vi "SCCSup OpenCloseFP.vi"(7 "function":enum16{"open FP", "close FP"}(ring), 8 "error in (no error)":errorcluster, 11 "VI Refnum in":refnum<vi>) -> (0 "error out":errorcluster, 3 "VI Refnum out":refnum<vi>)   [LabVIEW 2017]
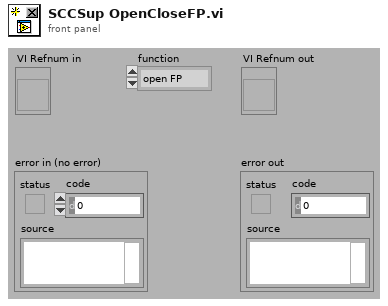
[diagram p1: front panel]
types:
  T1 = enum32{"Invalid", "Standard", "Closed", "Hidden", "Minimized", "Maximized"}
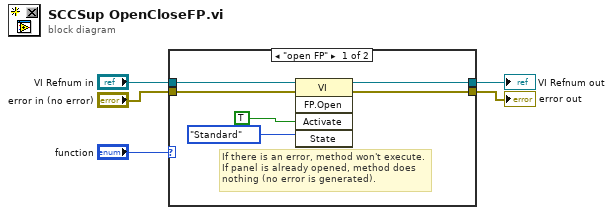
[diagram p0: block diagram]
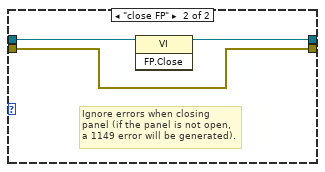
[diagram p2: hidden frame]
diagram:
  n1 = case shown="\"open FP\"" "function" {
    tunnel: "VI Refnum in" -> [w11 w14]
    tunnel: "error in (no error)" -> [w10 w13]
    tunnel: [w9 w13] -> w4
    tunnel: [w8 w12] -> w3
    frame "open FP" {
      # "If there is an error, method won't execute.  If panel is already opened, method does nothing (no error is generated)."
      n2 = invoke class="VI" method="FP.Open"(reference=w11, error in=w10, "Activate"=TRUE, "State"=T1."Standard") -> (reference out=w8:refnum<vi>, error out=w9:errorcluster)  [unwired: 1 in, 3 out]
    }
    frame "close FP" {
      # "Ignore errors when closing panel (if the panel is not open, a 1149 error will be generated)."
      n3 = invoke class="VI" method="FP.Close"(reference=w14) -> (reference out=w12:refnum<vi>)  [unwired: 2 in, 2 out]
    }
  }
  "error out" <- w4
  "VI Refnum out" <- w3
